vi "ParseCommand_Prepare_v2b.vi"(0 "1D functions":T6[](array[typedef]), 2 "Picture areas":T4[](array[typedef]), 3 "Command":string) -> (4 "Special Commands":T1[](array[typedef]), 5 "1D Assigned function":T5[](array[typedef]), 6 "2D Assigned function":T3[](array[typedef]), 7 "Temperature Assigned function":T2[](array[typedef]), 8 "Parsed command":string)   [LabVIEW 2010]
uses:
  Corrections.ctl
  PictureAreaControl.ctl
  1DAssignedFunction.ctl
  2DAssignedFunction.ctl
  TemperatureAssignedFunction.ctl
  SepcialCommands.ctl
panel:
  in  "Special Commands":T1[](array[typedef])
  in  "Special command":T1
  in  "Temperature Assigned function":T2[](array[typedef])
  in  "Temperature assigned function":T2
  in  "2D Assigned function":T3[](array[typedef])
  in  "2D assigned function":T3
  in  "1D Assigned function":T5[](array[typedef])
  in  "1D assigned function":T5
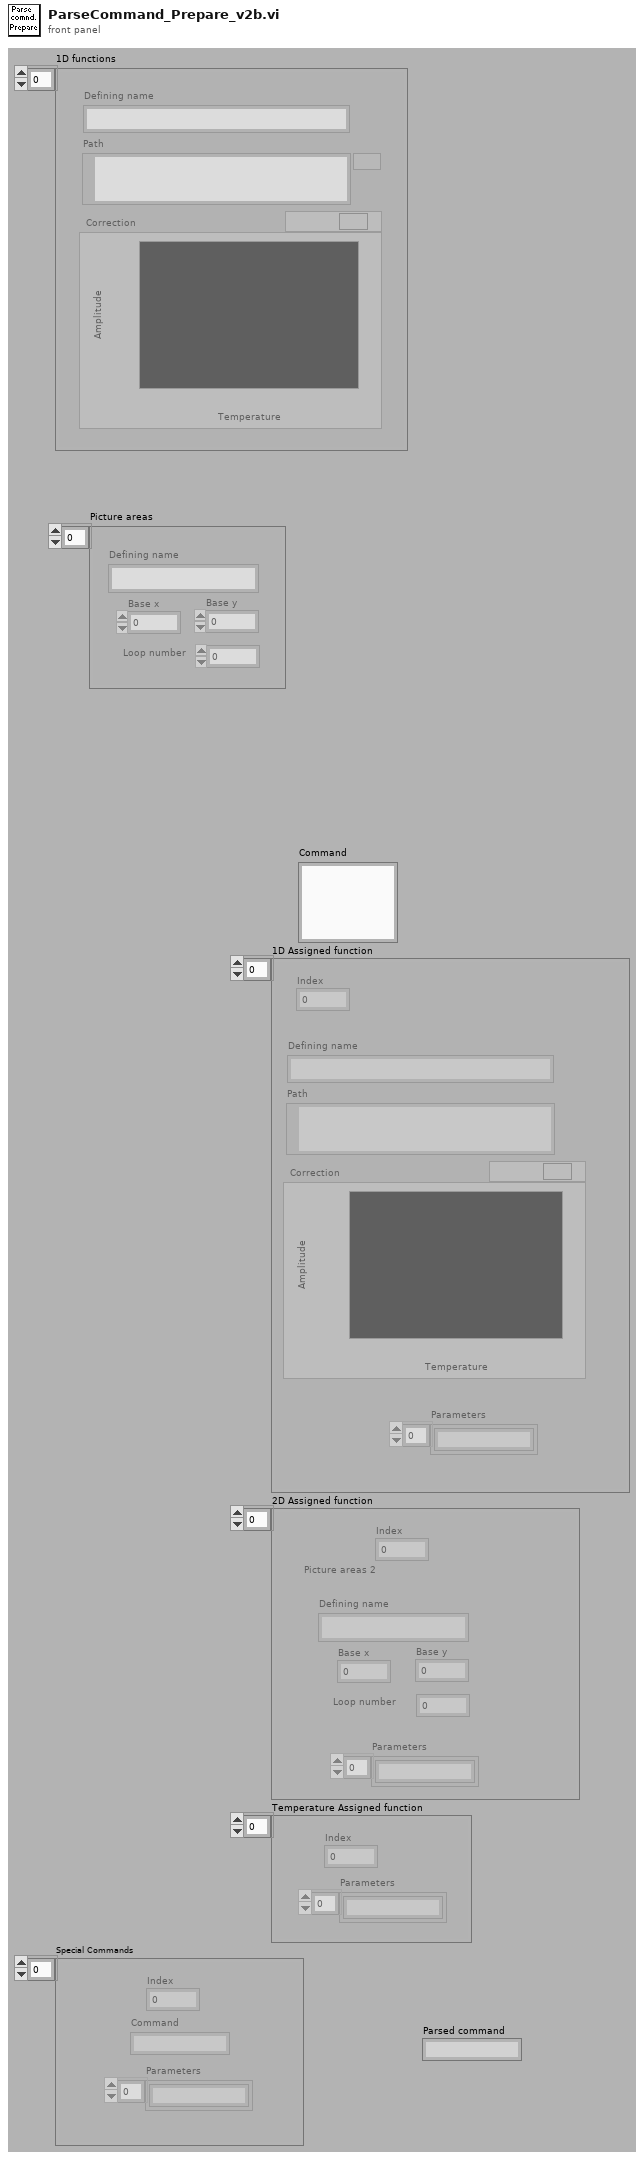
[diagram p1: front panel]
types:
  T1 = typedef "SepcialCommands.ctl" = cluster{"Index":dbl, "Command":string, "Parameters":string[]}
  T2 = typedef "TemperatureAssignedFunction.ctl" = cluster{"Index":dbl, "Parameters":string[]}
  T3 = typedef "2DAssignedFunction.ctl" = cluster{"Index":dbl, "Picture areas 2":T4, "Parameters":string[]}
  T4 = typedef "PictureAreaControl.ctl" = cluster{"Defining name":string, "Base x":dbl, "Base y":dbl, "Loop number":dbl}
  T5 = typedef "1DAssignedFunction.ctl" = cluster{"Index":dbl, "Corrections":T6, "Parameters":string[]}
  T6 = typedef "Corrections.ctl" = cluster{"Path":path, "Defining name":string, "Correction":cluster{dbl, dbl}[]}
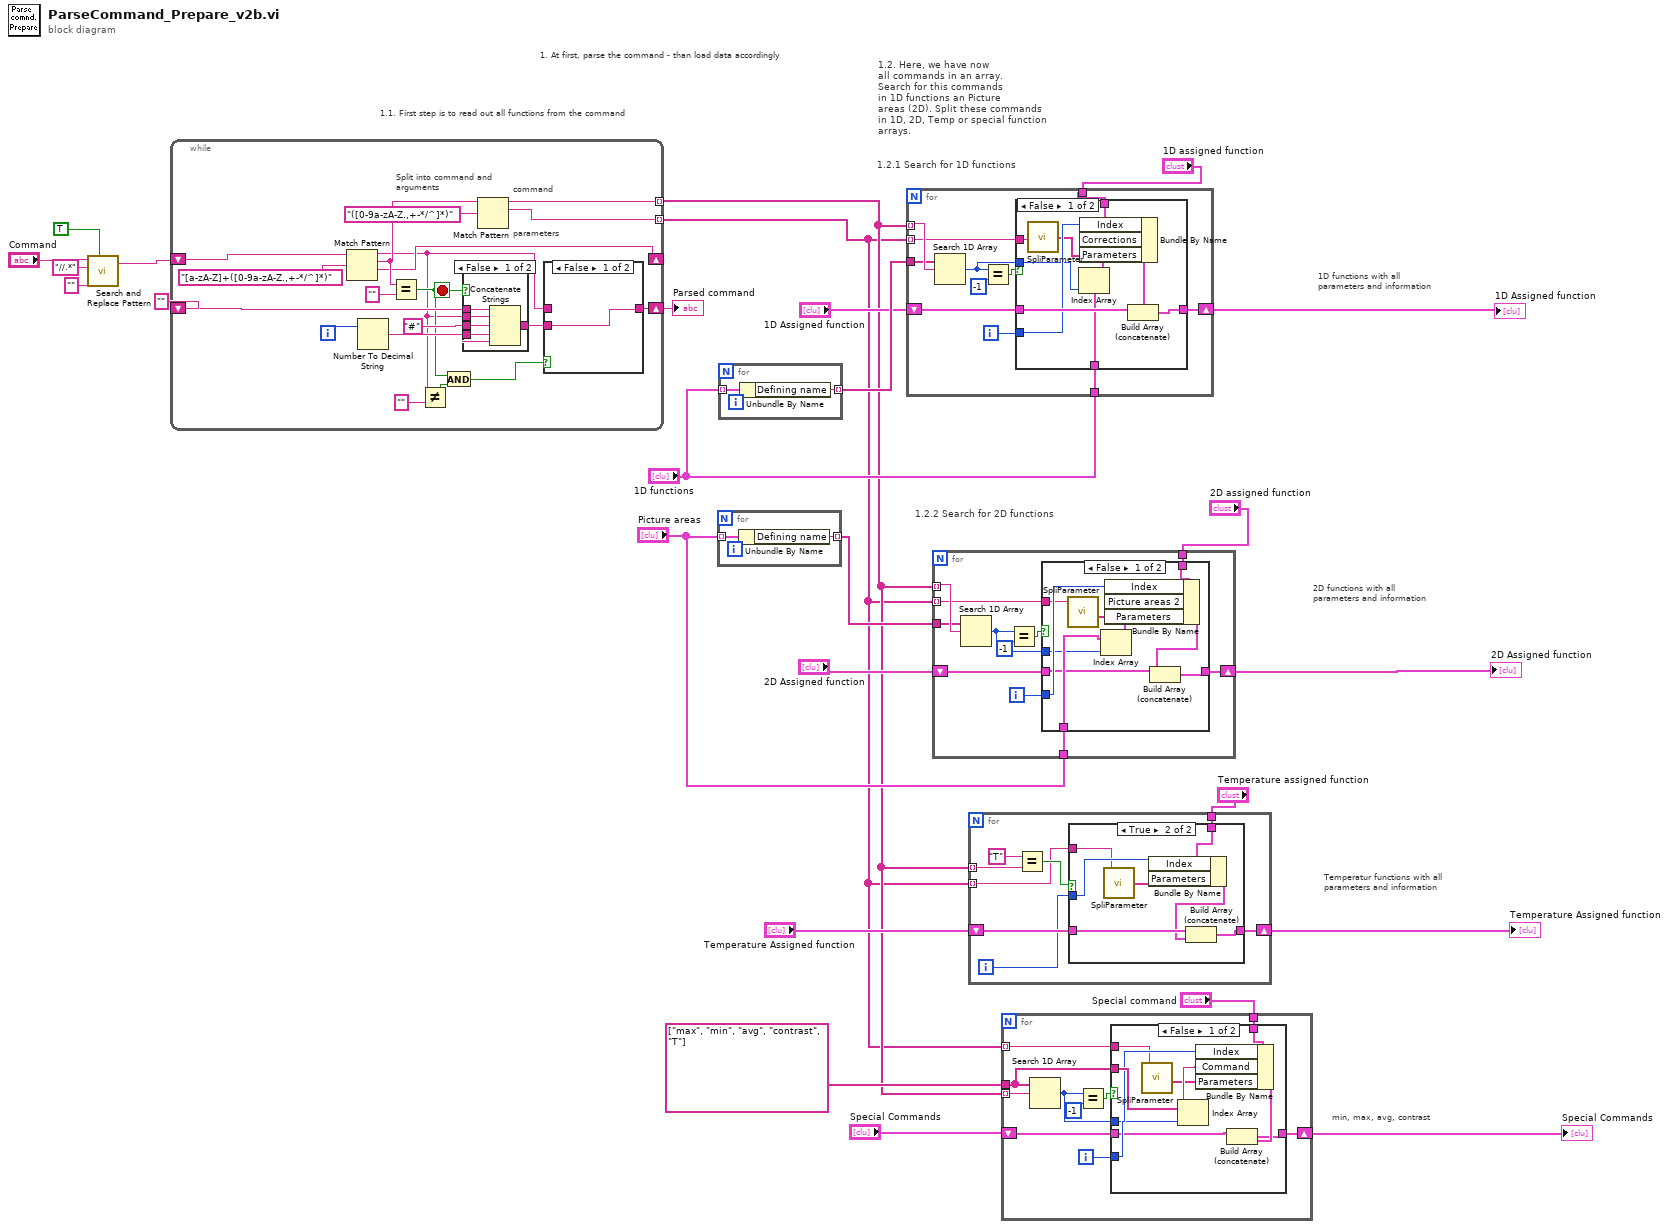
[diagram p0: block diagram]
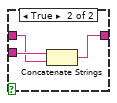
[diagram p5: hidden frame]
diagram:
  # "min, max, avg, contrast"
  # "Temperatur functions with all\nparameters and information"
  # "2D functions with all\nparameters and information"
  # "1.2.2 Search for 2D functions"
  # "1D functions with all\nparameters and information"
  # "1.2.1 Search for 1D functions"
  # "1.2. Here, we have now\nall commands in an array.\nSearch for this commands \nin 1D functions an Picture\nareas (2D). Split these commands \nin 1D, 2D, Temp or special function arrays."
  # "1.1. First step is to read out all functions from the command"
  # "1. At first, parse the command - than load data accordingly"
  n1 = call <vilib>:"Search and Replace Pattern.vi"("string"="Command", "regular expression (\"\")"="//.*" ("regular expression (\"\")"), "replace string (\"\")"="" ("replace string (\"\")"), "replace all? (F)"=TRUE) -> ("result string"=w4:string)  [unwired: 1 in, 1 out]
  n2 = while {
    shift-right: [w34] -> _
    shift-left: w4 -> [w45]
    tunnel: [w41] -> w12 mode=indexing
    tunnel: [w40] -> w10 mode=indexing
    shift-right: [w27] -> w6
    shift-left: "" -> [w38]
    i -> [w36]
    stop <- w31 stop-if-true
    # "command"
    # "parameters"
    # "Split into command and\narguments"
    n3 = Match Pattern(string=w45, regular expression="[a-zA-Z]+([0-9a-zA-Z.,+-*/^]*)") -> (before substring=w28:string, match substring=w39:string, after substring=w34:string)  [unwired: 1 in, 1 out]
    n4 = Number To Decimal String(number=w36) -> (decimal integer string=w35:string)  [unwired: 1 in]
    n5 = Equal?(x=w39, y="") -> (x = y?=w31:bool)
    n6 = Not Equal?(x=w28, y="") -> (x != y?=w32:bool)
    n7 = And(x=w31, y=w32) -> (x .and. y?=w30:bool)
    n8 = case shown="False" w31 {
      tunnel: w38 -> [w54 w55]
      tunnel: "#" ("string") -> [w53 _]
      tunnel: w35 -> [w52 _]
      tunnel: [w51 w55] -> w29
      tunnel: w28 -> [w50 _]
      frame False {
        n9 = Concatenate Strings(w54, w50, w53, w52, w53) -> (w51:string)
      }
      frame True {
      }
    }
    n10 = Match Pattern(string=w39, regular expression="([0-9a-zA-Z.,+-*/^]*)") -> (before substring=w41:string, match substring=w40:string)  [unwired: 1 in, 2 out]
    n11 = case shown="False" w30 {
      tunnel: w29 -> [w46 w49]
      tunnel: w28 -> [_ w48]
      tunnel: [w46 w47] -> w27
      frame False {
      }
      frame True {
        n12 = Concatenate Strings(w49, w48) -> (w47:string)
      }
    }
  }
  "Parsed command" <- w6
  n13 = for {
    tunnel: "Picture areas" -> [w57] mode=indexing
    tunnel: [w56] -> w22 mode=indexing
    n14 = Unbundle By Name(w57) -> ("Defining name"=w56:string)
  }
  n15 = for {
    tunnel: "1D functions" -> [w59] mode=indexing
    tunnel: [w58] -> w26 mode=indexing
    n16 = Unbundle By Name(w59) -> ("Defining name"=w58:string)
  }
  n17 = for {
    tunnel: w12 -> [w70] mode=indexing
    tunnel: w26 -> [w63]
    shift-right: [w67] -> w16
    shift-left: "1D Assigned function" -> [w68]
    tunnel: "1D assigned function" -> [w66]
    tunnel: "1D functions" -> [w62]
    tunnel: w10 -> [w61] mode=indexing
    i -> [w64]
    n18 = Search 1D Array(1D array=w63, element=w70) -> (index of element=w60:i32)  [unwired: 1 in]
    n19 = Equal?(x=w60, y=-1) -> (x = y?=w65:bool)
    n20 = case shown="False" w65 {
      tunnel: w68 -> [w80 w81]
      tunnel: [w79 w81] -> w67
      tunnel: w66 -> [w78 _]
      tunnel: w64 -> [w76 _]
      tunnel: w62 -> [w75 _]
      tunnel: w61 -> [w72 _]
      tunnel: w60 -> [w73 _]
      frame False {
        n21 = call "SpliParameter.vi"("Parameter"=w72) -> ("Output"=w71:string[])
        n22 = Index Array(array=w75, index=w73) -> (element=w74:T6)
        n23 = Bundle By Name(cluster=w78, "Index"=w76, "Corrections"=w74, "Parameters"=w71) -> (w77:T5)
        n24 = Build Array (concatenate)(w80, w77) -> (w79:T5[])
      }
      frame True {
      }
    }
  }
  "1D Assigned function" <- w16
  n25 = for {
    tunnel: w12 -> [w92] mode=indexing
    tunnel: w22 -> [w86]
    shift-right: [w89] -> w15
    shift-left: "2D Assigned function" -> [w90]
    tunnel: w10 -> [w85] mode=indexing
    tunnel: "2D assigned function" -> [w84]
    tunnel: "Picture areas" -> [w83]
    i -> [w87]
    n26 = Search 1D Array(1D array=w86, element=w92) -> (index of element=w82:i32)  [unwired: 1 in]
    n27 = Equal?(x=w82, y=-1) -> (x = y?=w88:bool)
    n28 = case shown="False" w88 {
      tunnel: w90 -> [w97 w103]
      tunnel: [w96 w103] -> w89
      tunnel: w87 -> [w99 _]
      tunnel: w85 -> [w94 _]
      tunnel: w84 -> [w102 _]
      tunnel: w83 -> [w101 _]
      tunnel: w82 -> [w95 _]
      frame False {
        n29 = call "SpliParameter.vi"("Parameter"=w94) -> ("Output"=w93:string[])
        n30 = Index Array(array=w101, index=w95) -> (element=w100:T4)
        n31 = Bundle By Name(cluster=w102, "Index"=w99, "Picture areas 2"=w100, "Parameters"=w93) -> (w98:T3)
        n32 = Build Array (concatenate)(w97, w98) -> (w96:T3[])
      }
      frame True {
      }
    }
  }
  "2D Assigned function" <- w15
  n33 = for {
    tunnel: w12 -> [w111] mode=indexing
    tunnel: w10 -> [w104] mode=indexing
    shift-right: [w107] -> w14
    shift-left: "Temperature Assigned function" -> [w108]
    tunnel: "Temperature assigned function" -> [w106]
    i -> [w105]
    n34 = Equal?(x="T", y=w111) -> (x = y?=w109:bool)
    n35 = case shown="True" w109 {
      tunnel: w108 -> [w112 w119]
      tunnel: [w112 w118] -> w107
      tunnel: w106 -> [_ w117]
      tunnel: w105 -> [_ w116]
      tunnel: w104 -> [_ w114]
      frame False {
      }
      frame True {
        n36 = call "SpliParameter.vi"("Parameter"=w114) -> ("Output"=w113:string[])
        n37 = Bundle By Name(cluster=w117, "Index"=w116, "Parameters"=w113) -> (w115:T2)
        n38 = Build Array (concatenate)(w119, w115) -> (w118:T2[])
      }
    }
  }
  "Temperature Assigned function" <- w14
  n39 = for {
    shift-right: [w127] -> w8
    shift-left: "Special Commands" -> [w128]
    tunnel: string[] ["max", "min", "avg", "contrast", "T"] ("Preused Strings") -> [w122]
    tunnel: w12 -> [w124] mode=indexing
    tunnel: "Special command" -> [w123]
    tunnel: w10 -> [w121] mode=indexing
    i -> [w125]
    n40 = Search 1D Array(1D array=w122, element=w124) -> (index of element=w120:i32)  [unwired: 1 in]
    n41 = Equal?(x=w120, y=-1) -> (x = y?=w126:bool)
    n42 = case shown="False" w126 {
      tunnel: w128 -> [w134 w140]
      tunnel: [w133 w140] -> w127
      tunnel: w125 -> [w136 _]
      tunnel: w123 -> [w139 _]
      tunnel: w122 -> [w138 _]
      tunnel: w121 -> [w131 _]
      tunnel: w120 -> [w132 _]
      frame False {
        n43 = call "SpliParameter.vi"("Parameter"=w131) -> ("Output"=w130:string[])
        n44 = Index Array(array=w138, index=w132) -> (element=w137:string)
        n45 = Bundle By Name(cluster=w139, "Index"=w136, "Command"=w137, "Parameters"=w130) -> (w135:T1)
        n46 = Build Array (concatenate)(w134, w135) -> (w133:T1[])
      }
      frame True {
      }
    }
  }
  "Special Commands" <- w8
